vi "sequencerHandshakes.vi"(11 "VoltOrScaler?":bool) -> ()   [LabVIEW 2014]
uses:
  <vilib>/Platform/TimedLoop/XDataNode/timing_clust.ctl
  <vilib>/Platform/TimedLoop/XDataNode/nitl_modes.ctl
  <vilib>/Platform/TimedLoop/XDataNode/wakeup.ctl
  <vilib>/rvi/Emulation/niFpgaSctlEmulationGetInTimedLoop.vi
  <vilib>/rvi/Emulation/niFpgaEmulationReportErrorSimple.vi
  <vilib>/rvi/Emulation/niFpgaGetClockAttributes.vi
  <vilib>/rvi/Emulation/niFpgaCriticalErrorInLSC.vi
  sequencerGlobVars.vi
  <vilib>/rvi/Emulation/niFpgaEmulationIsFPGAContextNoSignature.vi
  <vilib>/rvi/DataTransferAndStorage/Container/Common/niFpgaContainerGetUniqueNameForEmu.vi
  <vilib>/rvi/eio/common/nirviEmuReportErrorAndStop.vi
  <vilib>/rvi/Emulation/niFpgaProcessEmulError.vi
  <vilib>/Platform/TimedLoop/XDataNode/XDataNode.xnode
  <vilib>/rvi/DataTransferAndStorage/Container/XNode/niFpgaContainer.xnode
  <vilib>/rvi/DataTransferAndStorage/Handshake/Emulation/niFpgaHandshakeEmulation.vi
  <vilib>/Platform/TimedLoop/XDataNode/XDNodeRunTimeDep.lvlib
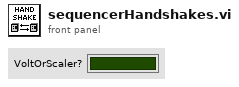
[diagram p1: front panel]
types:
  T1 = typedef "XDNodeRunTimeDep.lvlib/timing_clust.ctl" = cluster{"Expected End [f-1]":u64, "Actual End [f-1]":u64, "Finished Late? [f-1]":bool, "Expected End [i-1]":u64, "Actual End [i-1]":u64, "Finished Late? [i-1]":bool, "Expected Start [i]":u64, "Actual Start [i]":u64, "Expected Start [f]":u64, "Actual Start [f]":u64, "Source Name":string, "Structure Name":string, "Period":i64, "Deadline":i64, "Offset":i64, "Start":i64, "Priority":i32, "Timeout":i32, "Mode":T2, "Wakeup Reason":T3, "Error":errorcluster, "Source Type":string, "Secondary Source Type":string, "Global End Time":u64, "Global Start Time":u64, "Frame Duration":u64, "Iteration Duration":u64, "Assigned CPU":i32, "I/O Scan Engine Mode":u32}
  T2 = typedef "XDNodeRunTimeDep.lvlib/nitl_modes.ctl" = enum32{"No Change", "Process missed periods, maintain original phase", "Discard missed periods, maintain original phase", "Process missed periods, ignore original phase", "Discard missed periods, ignore original phase"}
  T3 = typedef "XDNodeRunTimeDep.lvlib/wakeup.ctl" = enum32{"Normal", "Aborted", "Asynchronous wakeup", "Timing source error", "Timed loop error", "Timeout"}
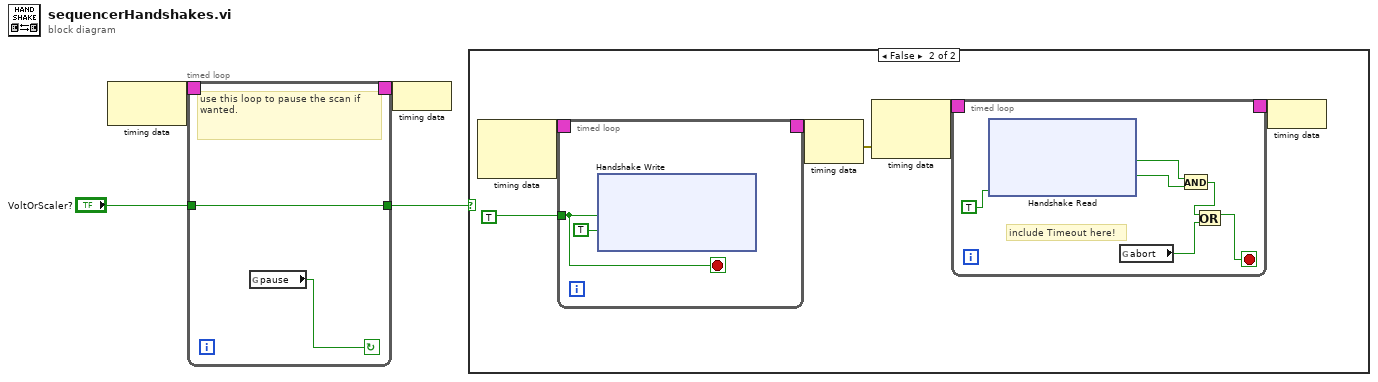
[diagram p0: block diagram]
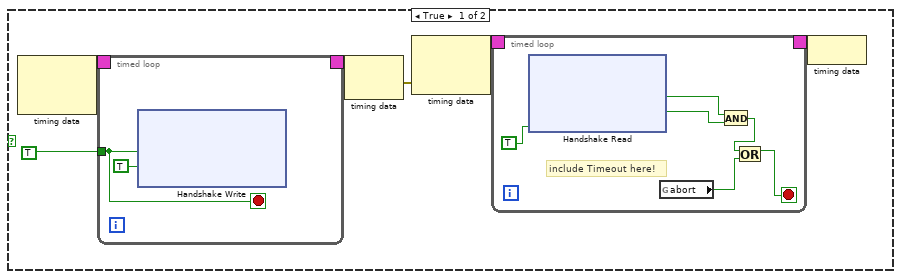
[diagram p2: hidden frame]
diagram:
  n1 = node-c288() -> (w4:T1)  [unwired: 1 in]
  n2 = timed-loop {
    timing: w4 -> [_]
    timing-out: [_] -> w3
    tunnel: [w6] -> w1
    tunnel: "VoltOrScaler?" -> [w6]
    stop <- w5 continue-if-true
    # "use this loop to pause the scan if wanted."
    n3 = global read "sequencerGlobVars.vi" "pause"() -> (w5:bool)
  }
  n4 = node-c288(w3) -> ()
  n5 = case shown="False" w1 {
    frame True {
      n6 = node-c288() -> (w14:T1)  [unwired: 2 in]
      n7 = timed-loop {
        timing: w14 -> [_]
        timing-out: [_] -> w13
        tunnel: TRUE -> [w27]
        stop <- w27 stop-if-true
        n8 = xnode ("Handshake Write")("Data"=w27, "Input Valid"=TRUE) -> ()  [unwired: 1 in, 2 out]
      }
      n9 = node-c288(w13) -> (w10:errorcluster)
      n10 = node-c288(w10) -> (w12:T1)  [unwired: 1 in]
      n11 = timed-loop {
        timing: w12 -> [_]
        timing-out: [_] -> w11
        stop <- w16 stop-if-true
        # "include Timeout here!"
        n12 = xnode ("Handshake Read")("Ready for Output"=TRUE) -> ("Data"=w19:bool, "Output Valid"=w18:bool)  [unwired: 1 in, 1 out]
        n13 = global read "sequencerGlobVars.vi" "abort"() -> (w15:bool)
        n14 = And(x=w19, y=w18) -> (x .and. y?=w20:bool)
        n15 = Or(x=w20, y=w15) -> (x .or. y?=w16:bool)
      }
      n16 = node-c288(w11) -> ()
    }
    frame False {
      n17 = node-c288() -> (w39:T1)  [unwired: 2 in]
      n18 = timed-loop {
        timing: w39 -> [_]
        timing-out: [_] -> w38
        tunnel: TRUE -> [w52]
        stop <- w52 stop-if-true
        n19 = xnode ("Handshake Write")("Data"=w52, "Input Valid"=TRUE) -> ()  [unwired: 1 in, 2 out]
      }
      n20 = node-c288(w38) -> (w35:errorcluster)
      n21 = node-c288(w35) -> (w37:T1)  [unwired: 1 in]
      n22 = timed-loop {
        timing: w37 -> [_]
        timing-out: [_] -> w36
        stop <- w41 stop-if-true
        # "include Timeout here!"
        n23 = xnode ("Handshake Read")("Ready for Output"=TRUE) -> ("Data"=w44:bool, "Output Valid"=w43:bool)  [unwired: 1 in, 1 out]
        n24 = global read "sequencerGlobVars.vi" "abort"() -> (w40:bool)
        n25 = And(x=w44, y=w43) -> (x .and. y?=w45:bool)
        n26 = Or(x=w45, y=w40) -> (x .or. y?=w41:bool)
      }
      n27 = node-c288(w36) -> ()
    }
  }
